vi "cfgSettings.vi"(6 "calConst":T4={"Cell 1"={"m"=1.0, "b"=0.0}, "Cell 2"={"m"=1.0, "b"=0.0}, "Cell 3"={"m"=1.0, "b"=0.0}, "Cell 4"={"m"=1.0, "b"=0.0}, "Cell 5"={"m"=1.0, "b"=0.0}} caption="Calibration Constants", 7 "Action":enum16{"Init", "Set", "Get"}(ring), 8 "SpkDutCyc":T3={"period"=150.0, "length"=2.0} caption="Speaker Duty Cycle", 9 "filtSet":T5={"sampPer"=300, "filtPer"=20} caption="Filter Duty Cycle", 11 "tauAnalysis":T1={"Red"=enum."LRS", "Blue"=enum."LRS", "Green"=enum."LRS"} caption="Exponential Fit \nMethod") -> (2 "CfgGood?":bool=TRUE)   [LabVIEW 2012]
uses:
  Controls/filtSetting.ctl
  Controls/expFitMethod.ctl
  Reusable/CRDS/Cell/Get Tau Method.ctl
  Controls/calConst.ctl
  Reusable/PAS/Main/Controls/period_length.ctl
  <userlib>/_JGCODE/error_logger/_error_logger.llb/ErrorLogger.lvclass
  Reusable/PAS/Base PAS.lvlib
  Shared Variables/PAS.lvlib
  Reusable/CRDS/Base CRDS Lib.lvlib
panel:
  in  "crd_PID_high":cluster{"P":sgl, "I":sgl, "D":sgl}={"P"=1.0, "I"=1.0, "D"=2.0} caption="PID Gains \n(High RH)"
  in  "crd_PID_med":cluster{"P":sgl, "I":sgl, "D":sgl}={"P"=1.0, "I"=0.8, "D"=2.0} caption="PID Gains \n(Med RH)"
  in  "pas_PID":cluster{"P":sgl, "I":sgl, "D":sgl}={"P"=5.0, "I"=1.0, "D"=2.0} caption="PID Gains"
  # "CRDS Parameters"
  # "PAS Parameters"
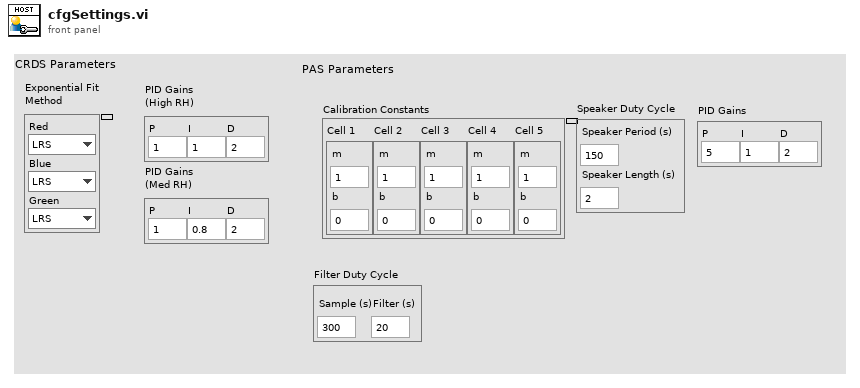
[diagram p1: front panel]
types:
  T1 = typedef "expFitMethod.ctl" = cluster{"Red":T2, "Blue":T2, "Green":T2}
  T2 = typedef "Base CRDS Lib.lvlib/Get Tau Method.ctl" = enum8{"DFT-1", "DFT-5", "LRS"}
  T3 = typedef "Base PAS.lvlib/period_length.ctl" = cluster{"period":sgl, "length":sgl}
  T4 = typedef "PAS.lvlib/calConst.ctl" = cluster{"Cell 1":cluster{"m":sgl, "b":sgl}, "Cell 2":cluster{"m":sgl, "b":sgl}, "Cell 3":cluster{"m":sgl, "b":sgl}, "Cell 4":cluster{"m":sgl, "b":sgl}, "Cell 5":cluster{"m":sgl, "b":sgl}}
  T5 = typedef "filtSetting.ctl" = cluster{"sampPer":u16, "filtPer":u16}
  T6 = cluster{"Array of Single[0]":sgl, "Array of Single[1]":sgl, "Array of Single[2]":sgl}
  T7 = cluster{"tauAnalysis":T1, "filtSet":T5, "SpkDutCyc":T3, "calConst":T4}
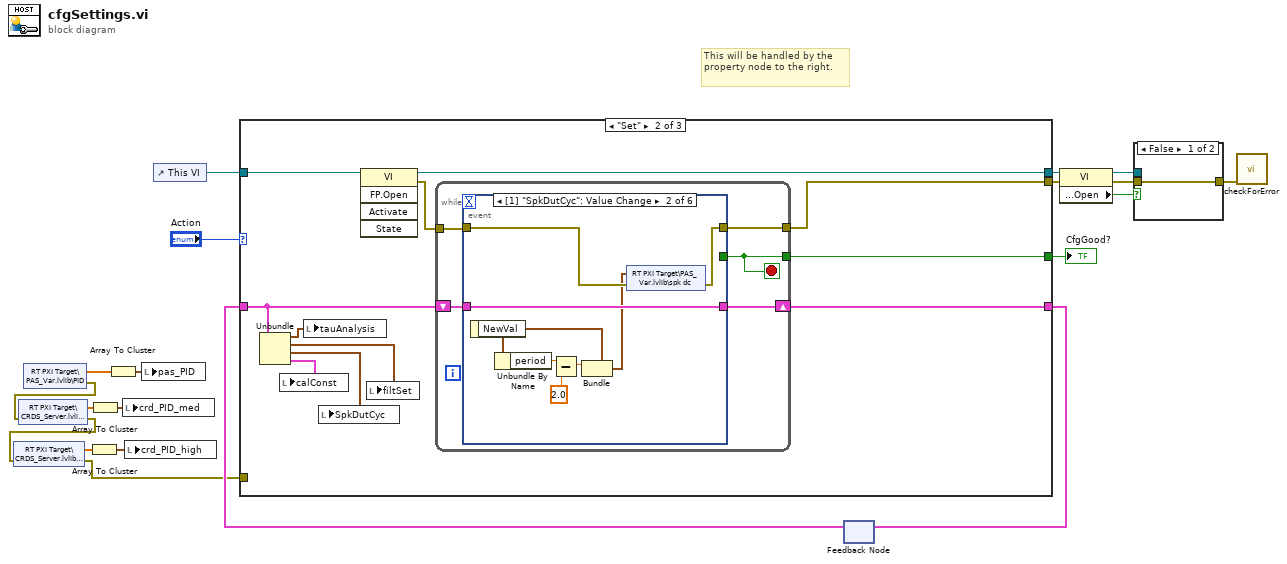
[diagram p0: block diagram]
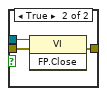
[diagram p2: hidden frame]
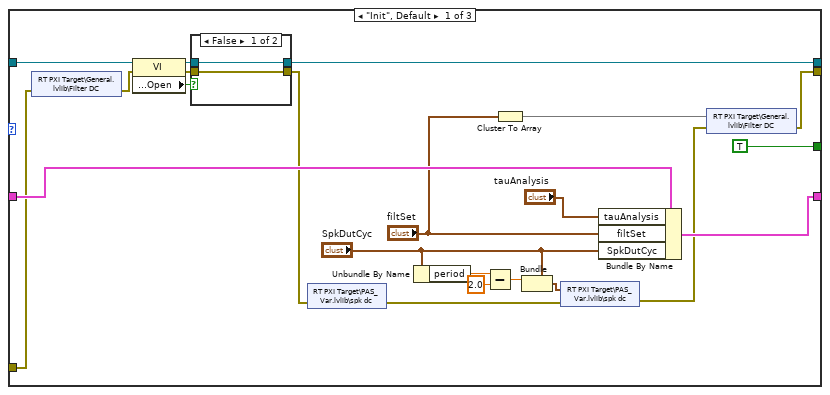
[diagram p3: hidden frame]
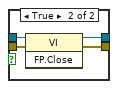
[diagram p4: hidden frame]
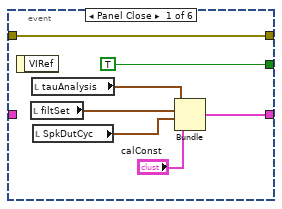
[diagram p5: hidden frame]
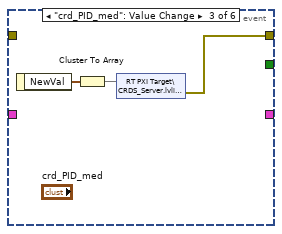
[diagram p6: hidden frame]
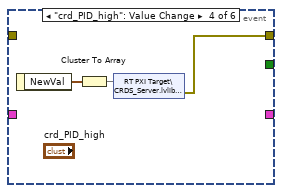
[diagram p7: hidden frame]
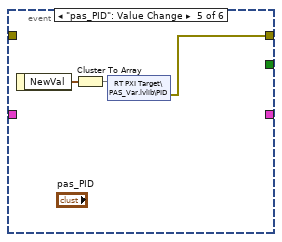
[diagram p8: hidden frame]
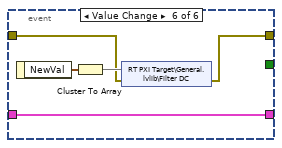
[diagram p9: hidden frame]
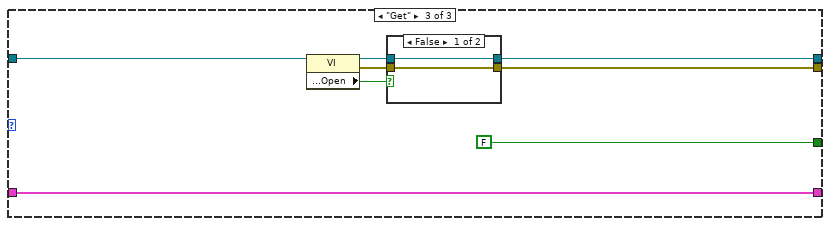
[diagram p10: hidden frame]
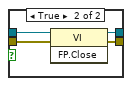
[diagram p11: hidden frame]
diagram:
  # "This will be handled by the property node to the right."
  n1 = shared-variable "RT PXI Target\\PAS_Var.lvlib\\PID"() -> (w9:sgl[], error out=w6:errorcluster)  [unwired: 1 in]
  n2 = shared-variable "RT PXI Target\\CRDS_Server.lvlib\\Med"(error in=w6) -> (w8:sgl[], error out=w3:errorcluster)
  n3 = shared-variable "RT PXI Target\\CRDS_Server.lvlib\\High"(error in=w3) -> (w4:sgl[], error out=w2:errorcluster)
  n4 = Array To Cluster(array=w4) -> (cluster=w5:T6)
  n5 = Array To Cluster(array=w8) -> (cluster=w7:T6)
  n6 = Array To Cluster(array=w9) -> (cluster=w10:T6)
  n7 = local write "crd_PID_med"(w7) -> ()
  n8 = local write "crd_PID_high"(w5) -> ()
  n9 = local write "pas_PID"(w10) -> ()
  n10 = control-ref of="This VI"() -> (w17:refnum<vi>)
  n11 = feedback #1() -> (w14:T7)  [unwired: 1 in]
  n12 = case shown="\"Set\"" "Action" {
    tunnel: [TRUE w59 FALSE] -> w20
    tunnel: [w22 w55 w97] -> w19
    tunnel: w17 -> [w41 w58 w98]
    tunnel: [w37 w57 w96] -> w16
    tunnel: [w35 w54 w94] -> w15
    tunnel: w14 -> [w36 w53 w94]
    tunnel: w2 -> [w21 _ _]
    frame "Init", Default {
      n13 = shared-variable "RT PXI Target\\General.lvlib\\Filter DC"(error in=w21) -> (error out=w25:errorcluster)  [unwired: 1 out]
      n14 = property class="VI"(reference=w41, error in=w25) -> (reference out=w40:refnum<vi>, error out=w39:errorcluster, "Front Panel.Open"=w38:bool)
      n15 = case shown="False" w38 {
        tunnel: w39 -> [w44 w48]
        tunnel: w40 -> [w43 w47]
        tunnel: [w44 w46] -> w24
        tunnel: [w43 w45] -> w37
        frame False {
        }
        frame True {
          n16 = invoke class="VI" method="FP.Close"(reference=w47, error in=w48) -> (reference out=w45:refnum<vi>, error out=w46:errorcluster)  [unwired: 1 in, 1 out]
        }
      }
      n17 = shared-variable "RT PXI Target\\PAS_Var.lvlib\\spk dc"(error in=w24) -> (error out=w34:errorcluster)  [unwired: 1 out]
      n18 = Unbundle By Name("SpkDutCyc") -> ("period"=w33:sgl)
      n19 = Subtract(x=w33, y=sgl 2.0) -> (x-y=w31:sgl)
      n20 = Cluster To Array(cluster="filtSet") -> (array=w27:u16[])
      n21 = Bundle(cluster="SpkDutCyc", "period"=w31) -> (w30:T3)  [unwired: 1 in]
      n22 = shared-variable "RT PXI Target\\PAS_Var.lvlib\\spk dc"(w30, error in=w34) -> (error out=w23:errorcluster)
      n23 = Bundle By Name(cluster=w36, "tauAnalysis"="tauAnalysis", "filtSet"="filtSet", "SpkDutCyc"="SpkDutCyc") -> (w35:T7)
      n24 = shared-variable "RT PXI Target\\General.lvlib\\Filter DC"(w27, error in=w23) -> (error out=w22:errorcluster)
    }
    frame "Set" {
      n25 = Unbundle(w53) -> ("tauAnalysis"=w52:T1, "filtSet"=w51:T5, "SpkDutCyc"=w50:T3, "calConst"=w49:T4)
      n26 = local write "calConst"(w49) -> ()
      n27 = local write "tauAnalysis"(w52) -> ()
      n28 = local write "SpkDutCyc"(w50) -> ()
      n29 = invoke class="VI" method="FP.Open"(reference=w58) -> (reference out=w57:refnum<vi>, error out=w56:errorcluster)  [unwired: 4 in, 3 out]
      n30 = local write "filtSet"(w51) -> ()
      n31 = while {
        tunnel: [w63] -> w59
        tunnel: w56 -> [w64]
        tunnel: [w62] -> w55
        shift-right: [w61] -> w54
        shift-left: w53 -> [w60]
        stop <- w63 stop-if-true
        n32 = event shown="[1] \"SpkDutCyc\": Value Change" {
          selector: _ -> [_ _ _ _ _ _]
          dyn-events: _ -> [_ _ _ _ _ _]
          timeout: _ -> [_ _ _ _ _ _]
          tunnel: [TRUE ("Discard?") _ _ _ _ _] -> w63
          tunnel: w64 -> [w69 w78 _ _ _ w91]
          tunnel: [w69 w79 w80 w83 w86 w90] -> w62
          tunnel: [w70 w77 _ _ _ w89] -> w61
          tunnel: w60 -> [_ w77 _ _ _ w89]
          event Panel Close {
            n33 = event-data() -> ()  [unwired: 1 in, 1 out]
            n34 = local read "filtSet"() -> (w67:T5)
            n35 = local read "tauAnalysis"() -> (w65:T1)
            n36 = local read "SpkDutCyc"() -> (w66:T3)
            n37 = Bundle("tauAnalysis"=w65, "filtSet"=w67, "SpkDutCyc"=w66, "calConst"="calConst") -> (w70:T7)  [unwired: 1 in]
          }
          event Value Change {
            n38 = event-data() -> ("NewVal"=w72:T3)  [unwired: 1 in]
            n39 = Unbundle By Name(w72) -> ("period"=w76:sgl)
            n40 = Subtract(x=w76, y=sgl 2.0) -> (x-y=w74:sgl)
            n41 = Bundle(cluster=w72, "period"=w74) -> (w73:T3)  [unwired: 1 in]
            n42 = shared-variable "RT PXI Target\\PAS_Var.lvlib\\spk dc"(w73, error in=w78) -> (error out=w79:errorcluster)
          }
          event "crd_PID_med": Value Change {
            n43 = event-data() -> ("NewVal"=w82:cluster{"P":sgl, "I":sgl, "D":sgl})  [unwired: 1 in]
            n44 = Cluster To Array(cluster=w82) -> (array=w81:sgl[])
            n45 = shared-variable "RT PXI Target\\CRDS_Server.lvlib\\Med"(w81) -> (error out=w80:errorcluster)  [unwired: 1 in]
          }
          event "crd_PID_high": Value Change {
            n46 = event-data() -> ("NewVal"=w85:cluster{"P":sgl, "I":sgl, "D":sgl})  [unwired: 1 in]
            n47 = Cluster To Array(cluster=w85) -> (array=w84:sgl[])
            n48 = shared-variable "RT PXI Target\\CRDS_Server.lvlib\\High"(w84) -> (error out=w83:errorcluster)  [unwired: 1 in]
          }
          event "pas_PID": Value Change {
            n49 = event-data() -> ("NewVal"=w88:cluster{"P":sgl, "I":sgl, "D":sgl})  [unwired: 1 in]
            n50 = Cluster To Array(cluster=w88) -> (array=w87:sgl[])
            n51 = shared-variable "RT PXI Target\\PAS_Var.lvlib\\PID"(w87) -> (error out=w86:errorcluster)  [unwired: 1 in]
          }
          event Value Change {
            n52 = event-data() -> ("NewVal"=w93:T5)  [unwired: 1 in]
            n53 = Cluster To Array(cluster=w93) -> (array=w92:u16[])
            n54 = shared-variable "RT PXI Target\\General.lvlib\\Filter DC"(w92, error in=w91) -> (error out=w90:errorcluster)
          }
        }
      }
    }
    frame "Get" {
      n55 = property class="VI"(reference=w98) -> (reference out=w101:refnum<vi>, error out=w100:errorcluster, "Front Panel.Open"=w99:bool)  [unwired: 1 in]
      n56 = case shown="False" w99 {
        tunnel: w100 -> [w103 w107]
        tunnel: w101 -> [w102 w106]
        tunnel: [w103 w105] -> w97
        tunnel: [w102 w104] -> w96
        frame False {
        }
        frame True {
          n57 = invoke class="VI" method="FP.Close"(reference=w106, error in=w107) -> (reference out=w104:refnum<vi>, error out=w105:errorcluster)  [unwired: 1 in, 1 out]
        }
      }
    }
  }
  "CfgGood?" <- w20
  n58 = feedback-in #1(w15) -> ()
  n59 = property class="VI"(reference=w16, error in=w19) -> (reference out=w12:refnum<vi>, error out=w11:errorcluster, "Front Panel.Open"=w13:bool)
  n60 = case shown="False" w13 {
    tunnel: w11 -> [w108 w111]
    tunnel: w12 -> [_ w110]
    tunnel: [w108 w109] -> w1
    frame False {
    }
    frame True {
      n61 = invoke class="VI" method="FP.Close"(reference=w110, error in=w111) -> (error out=w109:errorcluster)  [unwired: 1 in, 2 out]
    }
  }
  n62 = call <userlib>:"checkForError.vi"("Error In"=w1) -> ()  [unwired: 9 in, 2 out]
